vi "postToLabstepTimeline.vi"(7 "API Key":string, 8 "error in":errorcluster, 10 "Post contents":string, 11 "Post title":string) -> (0 "error out":errorcluster)   [LabVIEW 2018]
uses:
  <vilib>/httpClient/POSTBuffer.vi
  <vilib>/httpClient/LabVIEWHTTPClient.lvlib
panel:
  out "Server response debug panel":string
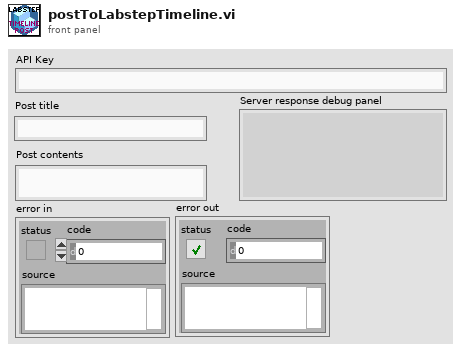
[diagram p1: front panel]
types:
  T1 = typedef "LabVIEWHTTPClient.lvlib/ClientHandle.ctl" = refnum<k1>
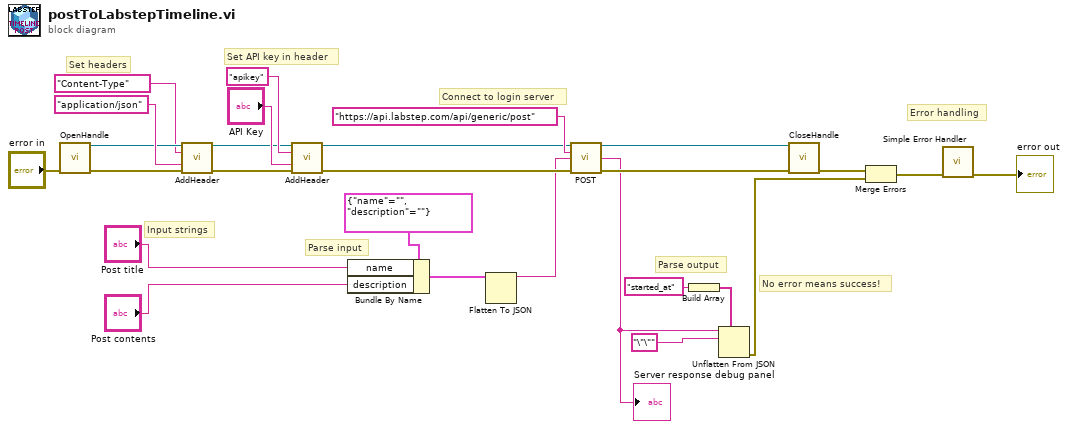
[diagram p0: block diagram]
diagram:
  # "Set API key in header"
  # "Error handling"
  # "Input strings"
  # "Set headers"
  # "Connect to login server"
  # "Parse input"
  # "No error means success!"
  # "Parse output"
  n1 = call <vilib>:"OpenHandle.vi"("error in (no error)"="error in") -> ("client handle out"=w23:T1, "error out"=w22:errorcluster)  [unwired: 13 in]
  n2 = call <vilib>:"AddHeader.vi"("client handle"=w23, "header"="Content-Type", "value"="application/json", "error in (no error)"=w22) -> ("client handle out"=w4:T1, "error out"=w7:errorcluster)  [unwired: 10 in]
  n3 = call <vilib>:"AddHeader.vi"("client handle"=w4, "header"="apikey", "value"="API Key", "error in (no error)"=w7) -> ("client handle out"=w5:T1, "error out"=w6:errorcluster)  [unwired: 10 in]
  n4 = Bundle By Name(cluster=cluster{"name":string, "description":string} {"name"="", "description"=""}, "name"="Post title", "description"="Post contents") -> (w21:cluster{"name":string, "description":string})
  n5 = Flatten To JSON(anything=w21) -> (JSON string=w1:string)  [unwired: 2 in, 1 out]
  n6 = call-poly <vilib>:"POST.vi"("client handle"=w5, "url"="https://api.labstep.com/api/generic/post", "buffer"=w1, "error in (no error)"=w6) -> ("client handle out"=w25:T1, "body"=w2:string, "error out"=w27:errorcluster)  [unwired: 8 in, 1 out]
  "Server response debug panel" <- w2
  n7 = Build Array("started_at") -> (w18:string[])
  n8 = Unflatten From JSON(path=w18, JSON string=w2, type and defaults="\"\"") -> (error out=w14:errorcluster)  [unwired: 4 in, 1 out]
  n9 = call <vilib>:"CloseHandle.vi"("client handle"=w25, "error in (no error)"=w27) -> ("error out"=w13:errorcluster)  [unwired: 13 in]
  n10 = Merge Errors(w13, w14) -> (w12:errorcluster)
  n11 = call <vilib>:"Simple Error Handler.vi"("error in (no error)"=w12) -> ("error out"=→"error out":errorcluster)  [unwired: 4 in, 4 out]
